vi "external trigger warning resonant.vi"(8 "queue ref in":refnum<queue>, 10 "FPGA VI Reference In":T1) -> ()   [LabVIEW 2012]
doc: "SciScan 1.2 160622"
uses:
  Custom Controls/FPGA reference typedef for 120MHz code.ctl
  Custom Controls/advanced settings inner tab CTL.ctl
  GFG/GFGbooleanGet.vi
  GFG/GFGfpRefGet.vi
  <vilib>/FPGAPlugInAG/Dynamic/niLvFpga_Abort_Dynamic.vi
  <vilib>/FPGAPlugInAG/Dynamic/niLvFpga_Close_Dynamic.vi
  <vilib>/rvi/interface/nirviMethod/nirviMethod.xnode
  <vilib>/rvi/interface/nirviCloseFPGA/nirviCloseFPGA.xnode
  GFG/GFG library.lvlib
panel:
  out "error out":errorcluster
  in  "stop 2":bool
  in  "String 3":string="WAITING FOR EXTERNAL TRIGGER"
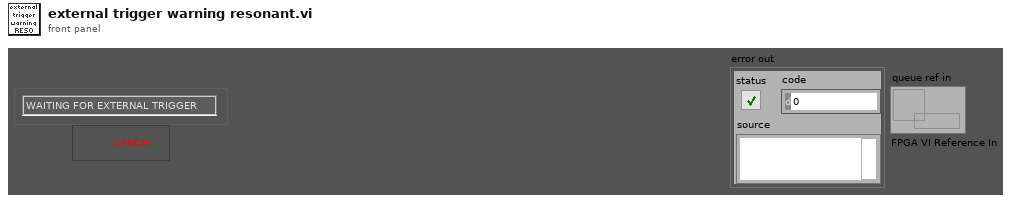
[diagram p1: front panel]
types:
  T1 = typedef "FPGA reference typedef for 120MHz code.ctl" = refnum<k20>
  T2 = enum32{"Invalid", "Default", "Floating", "Floating/Auto-Hide", "Modal"}
  T3 = enum32{"Invalid", "Standard", "Closed", "Hidden", "Minimized", "Maximized"}
  T4 = typedef "advanced settings inner tab CTL.ctl" = enum32{"arb. frames", "AO", "AI", "channels", "trigger", "Zstack data"}
  T5 = cluster{"WaveformChartRef":refnum<vi>, "DigitalRef":refnum<vi>, "ArrayRef":refnum<vi>, "TabControlRef":refnum<vi>, "EnumRef":refnum<vi>, "RingRef":refnum<vi>, "BooleanRef":refnum<vi>, "KnobRef":refnum<vi>, "SlideRef":refnum<vi>, "PathRef":refnum<vi>, "StringRef":refnum<vi>, "ComboBox":refnum<vi>, "WaveformGraphRef":refnum<vi>}
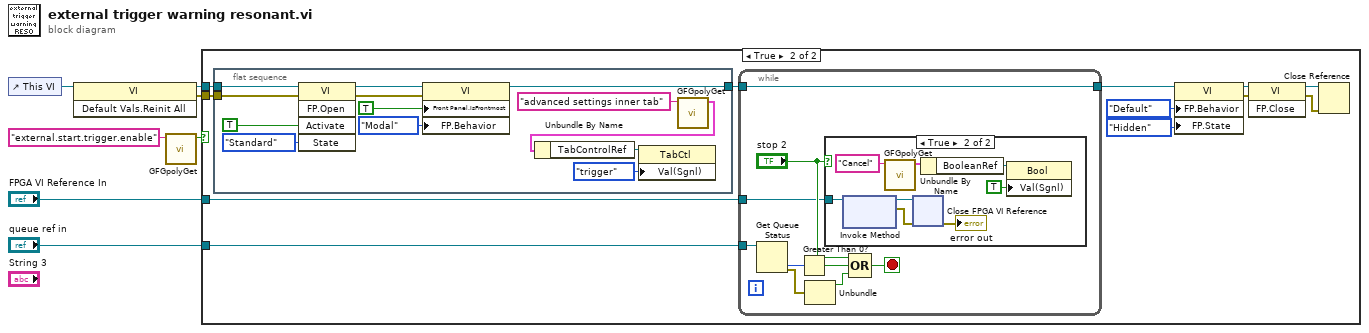
[diagram p0: block diagram]
diagram:
  n1 = control-ref of="This VI"() -> (w3:refnum<vi>)
  n2 = invoke class="VI" method="Default Vals.Reinit All"(reference=w3) -> (reference out=w2:refnum<vi>, error out=w1:errorcluster)  [unwired: 2 in, 1 out]
  n3 = call-poly "GFGpolyGet.vi"("Variable Name in"="external.start.trigger.enable" ("Tag in")) -> ("Boolean Value OUT"=w6:bool)  [unwired: 9 in, 1 out]
  n4 = case shown="True" w6 {
    tunnel: w2 -> [_ w19]
    tunnel: "queue ref in" -> [_ w18]
    tunnel: "FPGA VI Reference In" -> [_ w15]
    tunnel: w1 -> [_ w8]
    frame False {
    }
    frame True {
      n5 = flat-sequence {
        tunnel: w19 -> [w20]
        tunnel: [w26] -> w17
        tunnel: w8 -> [w21]
        frame #0 {
          n6 = invoke class="VI" method="FP.Open"(reference=w20, error in=w21, "Activate"=TRUE ("Activate?"), "State"=T3."Standard" ("Front Panel Window:State")) -> (reference out=w25:refnum<vi>, error out=w24:errorcluster)  [unwired: 1 in, 3 out]
          n7 = property class="VI"(reference=w25, error in=w24, "Front Panel.IsFrontmost"=TRUE ("Front Panel Window:Is Frontmost"), "FP.Behavior"=T2."Modal" ("Front Panel Window:Behavior")) -> (reference out=w26:refnum<vi>)  [unwired: 1 out]
          n8 = call-poly "GFGpolyGet.vi"("Variable Name in"="advanced settings inner tab") -> ("output cluster"=w30:T5)  [unwired: 9 in, 1 out]
          n9 = Unbundle By Name(w30) -> ("TabControlRef"=w29:refnum<vi>)
          n10 = property class="TabCtl"(reference=w29, "Val(Sgnl)"=advanced_settings_inner_tab_CTL."trigger" ("advanced settings inner tab")) -> ()  [unwired: 1 in, 2 out]
        }
      }
      n11 = while {
        tunnel: w18 -> [w41]
        tunnel: w17 -> [w36]
        tunnel: [w36] -> w16
        tunnel: w15 -> [w35]
        stop <- w38 stop-if-true
        n12 = Get Queue Status(queue=w41) -> (error out=w34:errorcluster, # elements in queue=w40:i32)  [unwired: 2 in, 6 out]
        n13 = Greater Than 0?(x=w40) -> (x > 0?=w39:bool)
        n14 = Unbundle(w34) -> ("status"=w33:bool)  [unwired: 2 out]
        n15 = case shown="True" "stop 2" {
          tunnel: w35 -> [_ w42]
          frame False {
          }
          frame True {
            n16 = xnode "Invoke Method"("FPGA VI Reference In"=w42) -> ("FPGA VI Reference Out"=w45:T1, "error out"=w44:errorcluster)  [unwired: 1 in]
            n17 = call-poly "GFGpolyGet.vi"("Variable Name in"="Cancel") -> ("output cluster"=w47:T5)  [unwired: 9 in, 1 out]
            n18 = xnode "Close FPGA VI Reference"("FPGA VI Reference In"=w45, "error in"=w44) -> ("error out"=→"error out":errorcluster)
            n19 = Unbundle By Name(w47) -> ("BooleanRef"=w48:refnum<vi>)
            n20 = property class="Bool"(reference=w48, "Val(Sgnl)"=TRUE ("Visible")) -> ()  [unwired: 1 in, 2 out]
          }
        }
        n21 = Compound Arithmetic op=OR("stop 2", w39, w33) -> (w38:bool)
      }
      n22 = property class="VI"(reference=w16, "FP.Behavior"=T2."Default" ("Front Panel Window:Behavior"), "FP.State"=T3."Hidden" ("Front Panel Window:State")) -> (reference out=w12:refnum<vi>, error out=w11:errorcluster)  [unwired: 1 in]
      n23 = invoke class="VI" method="FP.Close"(reference=w12, error in=w11) -> (reference out=w10:refnum<vi>, error out=w9:errorcluster)  [unwired: 1 in, 1 out]
      n24 = Close Reference(reference=w10, error in (no error)=w9) -> ()  [unwired: 1 out]
    }
  }
